vi "Update Card Position.vi"(7 "Card Position Ref":refnum<vi>, 8 "error in (no error)":errorcluster, 9 "NewVal":T2 {"Slot #" max=15}, 10 "OldVal":T2 {"Slot #" max=15}, 11 "Node Ptr in":T1 format="%.0x") -> (0 "error out":errorcluster)   [LabVIEW 2014, in "SLSC configuration System Explorer.lvlib"]
uses:
  SLSC configuration System Explorer.lvlib
  Type Defs/Card Position.ctl
  Shared/SPI Utility/Slot #.ctl
  <vilib>/NI Veristand/Custom Device API/Custom Device Item Ref.ctl
  Shared/Constants.vi
  Shared/SLSC configuration Shared.lvlib
  <vilib>/NI Veristand/Custom Device API/Custom Device API.lvlib
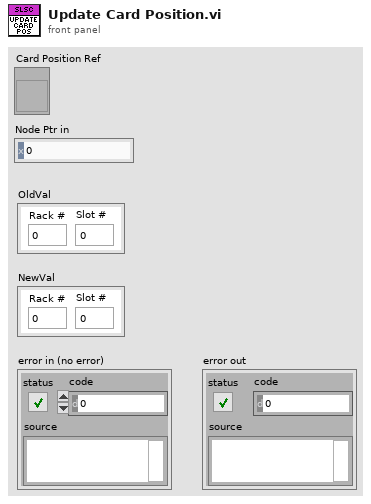
[diagram p1: front panel]
types:
  T1 = typedef "Custom Device API.lvlib/Custom Device Item Ref.ctl" = u64
  T2 = typedef "SLSC configuration Shared.lvlib/Card Position.ctl" = cluster{"Rack #":u8, "Slot #":T3}
  T3 = typedef "SLSC configuration Shared.lvlib/Slot #.ctl" = u8
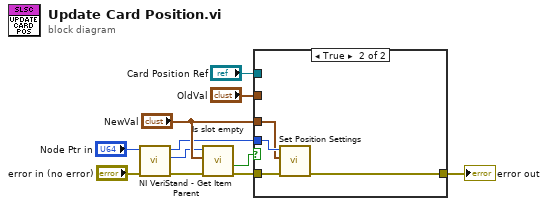
[diagram p0: block diagram]
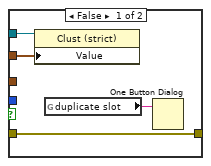
[diagram p2: hidden frame]
diagram:
  n1 = call <vilib>:"NI VeriStand - Get Item Parent.vi"("error in (no error)"="error in (no error)", "Item Ref in"="Node Ptr in") -> ("error out"=w7:errorcluster, "Parent Ref"=w6:T1, "Item Ref out"=w8:T1)  [unwired: 6 in, 1 out]
  n2 = call "Is slot empty.vi"("error in (no error)"=w7, "Card Position"="NewVal", "Devcie Ref in"=w6) -> ("error out"=w2:errorcluster, "Empty?"=w3:bool)  [unwired: 6 in, 1 out]
  n3 = case shown="True" w3 {
    tunnel: w2 -> [w14 w19]
    tunnel: [w14 w18] -> w4
    tunnel: w8 -> [_ w17]
    tunnel: "NewVal" -> [_ w16]
    tunnel: "OldVal" -> [w13 _]
    tunnel: "Card Position Ref" -> [w12 _]
    frame False {
      n4 = property class="Clust (strict)"(reference=w12, "Value"=w13) -> ()  [unwired: 1 in, 2 out]
      n5 = global read "Constants.vi" "duplicate slot"() -> (w15:string)
      n6 = One Button Dialog(message=w15) -> ()  [unwired: 1 in, 1 out]
    }
    frame True {
      n7 = call "Set Position Settings.vi"("error in (no error)"=w19, "Card Position"=w16, "Item Ref in"=w17) -> ("error out"=w18:errorcluster)  [unwired: 7 in, 1 out]
    }
  }
  "error out" <- w4
